vi "Control_DeInit_Done.vi"(8 "error in (no error)":errorcluster, 11 "Camera_Scan_Controller in":refnum<class "Camera_Scan_Controller.lvclass">) -> (0 "error out":errorcluster, 3 "Camera_Scan_Controller out":refnum<class "Camera_Scan_Controller.lvclass">)   [LabVIEW 2023, in "Camera_Scan_Controller.lvlib" / "Camera_Scan_Controller.lvclass"]
uses:
  Camera_Scan_Controller.lvclass
  Camera_Scan_Controller.lvclass/Camera_Scan_Controller.ctl
  <vilib>/ActorFramework/Message Enqueuer/Message Enqueuer.lvclass/Message Enqueuer.ctl
  <vilib>/ActorFramework/Message Enqueuer/Enqueue.vi
  <vilib>/ActorFramework/Stop Msg/Stop Msg.lvclass
  C:/Program Files/National Instruments/LabVIEW 2023/vi.lib/ActorFramework/Message/Message.lvclass
  <vilib>/ActorFramework/Message Priority Queue/Priority Enqueue.vi
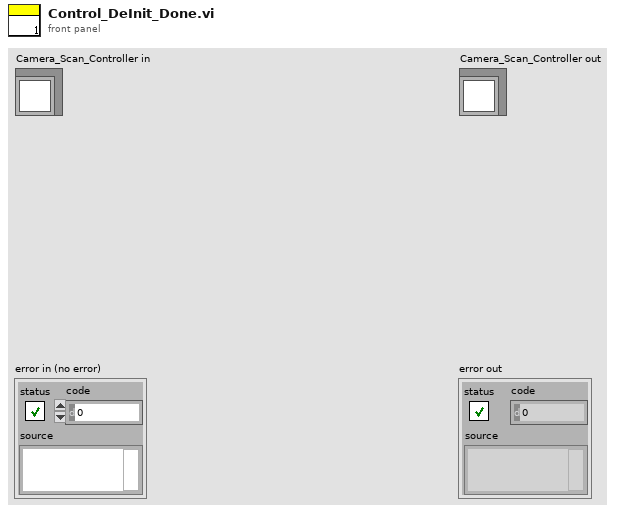
[diagram p1: front panel]
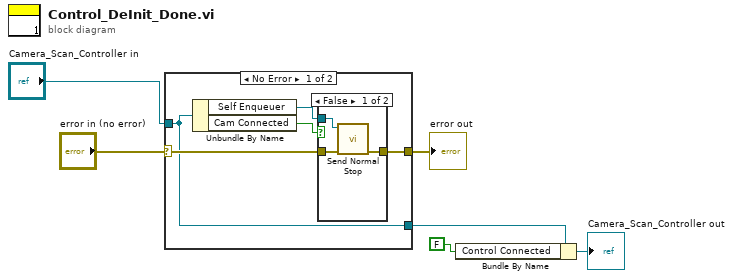
[diagram p0: block diagram]
diagram:
  n1 = case shown="No Error" "error in (no error)" {
    selector: "error in (no error)" -> [w9 w16]
    tunnel: "Camera_Scan_Controller in" -> [w8 w17]
    tunnel: [w10 w16] -> w2
    tunnel: [w8 w17] -> w6
    frame No Error {
      n2 = Unbundle By Name(w8) -> ("Self Enqueuer"=w7:refnum<class "Message Enqueuer.lvclass">, "Cam Connected"=w11:bool)
      n3 = case shown="False" w11 {
        tunnel: w9 -> [w14 w15]
        tunnel: [w13 w15] -> w10
        tunnel: w7 -> [w12 _]
        frame False {
          n4 = call <vilib>:"Send Normal Stop.vi"("error in (no error)"=w14, "Message Enqueuer"=w12) -> ("error out"=w13:errorcluster)  [unwired: 9 in]
        }
        frame True {
        }
      }
    }
    frame Error {
    }
  }
  "error out" <- w2
  n5 = Bundle By Name(cluster=w6, "Control Connected"=FALSE ("Cam Connected")) -> (→"Camera_Scan_Controller out":refnum<class "Camera_Scan_Controller.lvclass">)
